vi "CMD_04_set_Sending_flag.vi"(11 "Sending Flag":bool) -> ()   [LabVIEW 2017]
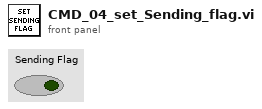
[diagram p1: front panel]
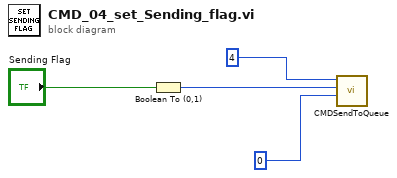
[diagram p0: block diagram]
diagram:
  n1 = Boolean To (0,1)(Boolean="Sending Flag") -> (0, 1=w1:i16)
  n2 = call "CMDSendToQueue.vi"("arg2"=i16 0, "arg1"=w1, "CMD"=i8 4) -> ()  [unwired: 9 in]
